vi "Configure Multi Eval Meas Spectrum ACLR Statistic Count.vi"(8 "error in (no error)":errorcluster, 9 "ACLR Statistic Count (20)":i32=20, 10 "Instance (1)":T1=1, 11 "VISA resource name":refnum<visa-resource-name>) -> (0 "error out":errorcluster, 3 "VISA resource name out":refnum<visa-resource-name>)   [LabVIEW 2020, in "Rohde&Schwarz CMWXP NR FR1 Measurement.lvlib"]
doc: "Specifies the statistic count of the measurement. The statistic count is equal to the number of measurement intervals per single shot.\nSeparate statistic counts for ACLR and spectrum emission mask measurements are supported.\n\nAttribute:\nRSCMWXPNRFR1M_ATTR_MULTI_EVAL_MEAS_SPECTRUM_ACLR_STATISTIC_COUNT\n\nRemote-control command:\nCONFigure:NRSub:MEAS<i>:MEValuation:SCOunt:SPECtrum:ACLR"
uses:
  <instrlib>/Rohde&Schwarz CMWXP NR FR1 Measurement/Rohde&Schwarz CMWXP NR FR1 Measurement.lvlib
  <instrlib>/Rohde&Schwarz CMWXP NR FR1 Measurement/Private/_Instance.ctl
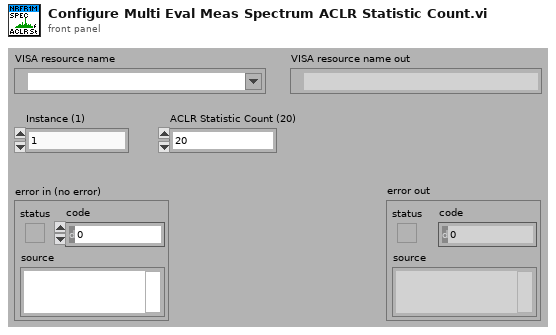
[diagram p1: front panel]
types:
  T1 = typedef "Rohde&Schwarz CMWXP NR FR1 Measurement.lvlib/_Instance.ctl" = i32
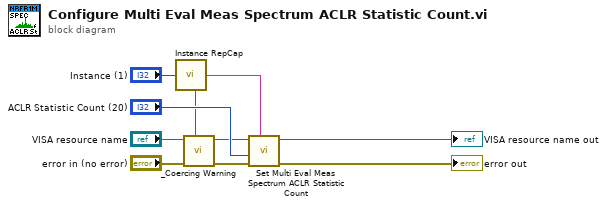
[diagram p0: block diagram]
diagram:
  n1 = call <instrlib>:"Instance RepCap.vi"("Instance In"="Instance (1)") -> ("In Range?"=w1:bool, "RepCap Identifier Out"=w7:string)  [unwired: 1 in]
  n2 = call <instrlib>:"_Coercing Warning.vi"("In Range?"=w1, "error in (no error)"="error in (no error)", "VISA resource name"="VISA resource name") -> ("error out"=w3:errorcluster, "VISA resource name out"=w2:refnum<visa-resource-name>)  [unwired: 7 in]
  n3 = call "Set Multi Eval Meas Spectrum ACLR Statistic Count"("Repeated Capabilities"=w7, "error in (no error)"=w3, "Multi Eval Meas Spectrum ACLR Statistic Count (0)"="ACLR Statistic Count (20)", "instrument handle"=w2) -> ("error out"=→"error out":errorcluster, "instrument handle out"=→"VISA resource name out":refnum<visa-resource-name>)  [unwired: 6 in]
